vi "UpdateMatlabDataValueToVartiant.vi"(9 "name":string, 10 "MatlabDataBundle":T1, 11 "Type (or value to update)":variant) -> (3 "Value":variant)   [LabVIEW 2017]
uses:
  Types/MatlabDataBundle.ctl
  Types/MatlabDataType.ctl
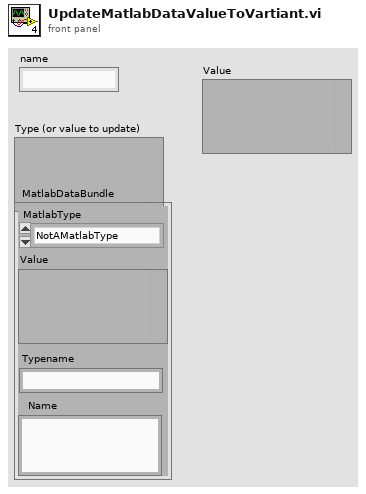
[diagram p1: front panel]
types:
  T1 = typedef "MatlabDataBundle.ctl" = cluster{"MatlabType":T2, "Value":variant, "Name":string, "Typename":string}
  T2 = typedef "MatlabDataType.ctl" = enum16{"NotAMatlabType", "Real", "Complex", "String", "Boolean"}
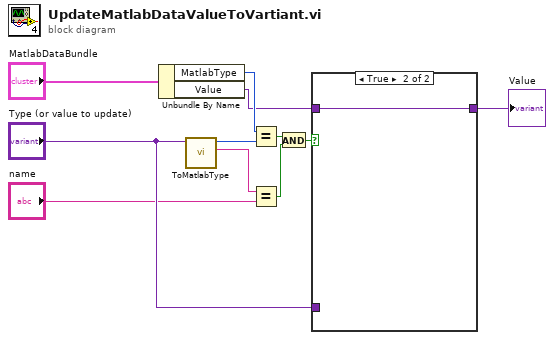
[diagram p0: block diagram]
diagram:
  n1 = Unbundle By Name("MatlabDataBundle") -> ("MatlabType"=w9:T2, "Value"=w5:variant)
  n2 = call "ToMatlabType.vi"("Value"="Type (or value to update)") -> ("Name"=w11:string, "MatlabType"=w10:T2)  [unwired: 7 in, 2 out]
  n3 = Equal?(x=w9, y=w10) -> (x = y?=w7:bool)
  n4 = Equal?(x=w11, y="name") -> (x = y?=w6:bool)
  n5 = And(x=w7, y=w6) -> (x .and. y?=w2:bool)
  n6 = case shown="True" w2 {
    tunnel: "Type (or value to update)" -> [w12 _]
    tunnel: [w12 w13] -> w3
    tunnel: w5 -> [_ w13]
    frame False {
    }
    frame True {
    }
  }
  "Value" <- w3
